vi "Read encoder velocity mMc.vi"(1 "Port":T1={"P type"=0, "reference"="", " Terminator "="\r\n", "Timeout"=300} {"Timeout" step=10; "P type" items=["none", "RS-232C"]}, 3 "error in (no error)":errorcluster, 5 "Controller #":string) -> (6 "Enc vel":dbl caption="Encoder velocity", 9 "error out":errorcluster)   [LabVIEW 2015]
doc: "VRT 命令：读取编码器速度"
panel:
  # "Read encoder velocity"
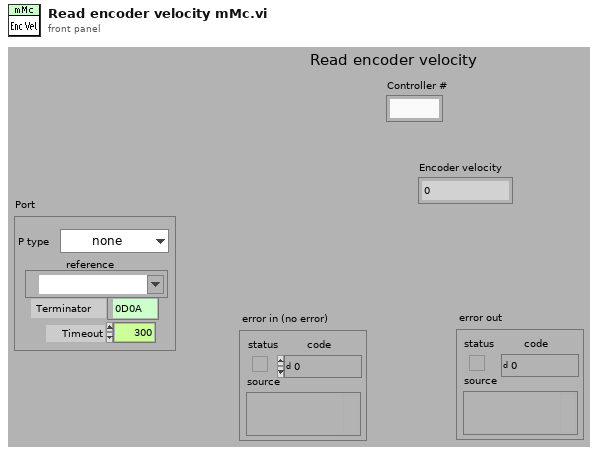
[diagram p1: front panel]
types:
  T1 = cluster{"P type":u16, "reference":refnum<visa-resource-name>, " Terminator ":string, "Timeout":i32}
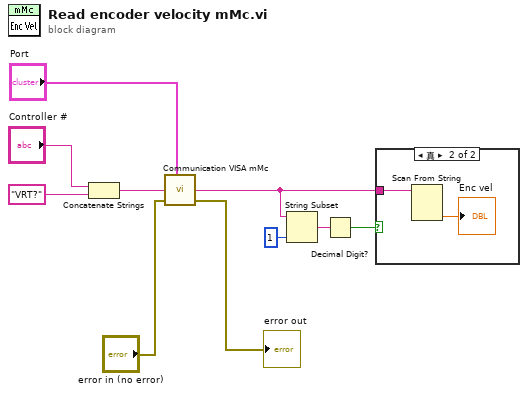
[diagram p0: block diagram]
diagram:
  n1 = Concatenate Strings("Controller #", "VRT?") -> (w6:string)
  n2 = call <instrlib>:"Communication VISA mMc.vi"("Port"="Port", "Command"=w6, "error in (no error)"="error in (no error)") -> ("Return"=w1:string, "error out"=→"error out":errorcluster)  [unwired: 3 in, 2 out]
  n3 = String Subset(string=w1, length (rest)=1 ("length (rest)")) -> (substring=w3:string)  [unwired: 1 in]
  n4 = Decimal Digit?(1:w3) -> (0:w2:bool)
  n5 = case shown="真" w2 {
    tunnel: w1 -> [_ w11]
    frame False {
    }
    frame True {
      n6 = Scan From String(input string=w11) -> (output 1=→"Enc vel":dbl)  [unwired: 4 in, 3 out]
    }
  }
